vi "Write_Register.vi"(8 "error in (no error)":errorcluster, 9 "Value":u16, 10 "Address":u16 format="%x", 11 "Serial Config":T1={"Baud"=9600, "Flow Ctl"=0, "Parity"=0, "Address"=1, "VISA resource name"=""} {"Parity" items=["None", "Odd", "Even"]; "Flow Ctl" items=["None"]; "Baud" items=["4800"=4800, "9600"=9600, "19200"=19200, "38400"=38400]}) -> (0 "error out":errorcluster, 3 "Serial Config out":T1={"Baud"=9600, "Flow Ctl"=0, "Parity"=0, "Address"=0, "VISA resource name"=""} {"Parity" items=["None", "Odd", "Even"]; "Flow Ctl" items=["None"]; "Baud" items=["4800"=4800, "9600"=9600, "19200"=19200, "38400"=38400]})   [LabVIEW 2014, in "Omega CN9600 series.lvclass"]
uses:
  Omega CN9600 series.lvclass
  Serial_Config_Omega.ctl
  <vilib>/Utility/error.llb/Error Cluster From Error Code.vi
  <vilib>/ErrorRing/Error Ring.xnode
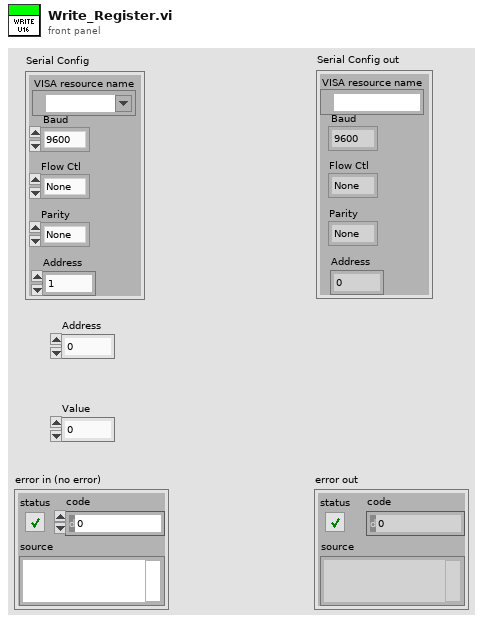
[diagram p1: front panel]
types:
  T1 = typedef "Omega CN9600 series.lvclass/Serial_Config_Omega.ctl" = cluster{"Baud":u32, "Flow Ctl":u16, "Parity":u16, "Address":u8, "VISA resource name":refnum<visa-resource-name>}
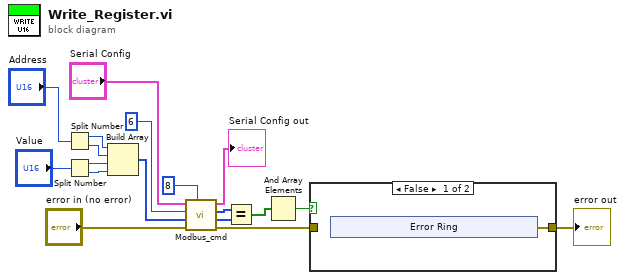
[diagram p0: block diagram]
diagram:
  n1 = Split Number(x="Address") -> (hi(x)=w12:u8, lo(x)=w11:u8)
  n2 = Split Number(x="Value") -> (hi(x)=w2:u8, lo(x)=w1:u8)
  n3 = Build Array(w12, w11, w2, w1) -> (w10:u8[])
  n4 = call "Modbus_cmd.vi"("Bytes to read"=u32 8, "error in (no error)"="error in (no error)", "Data"=w10, "Function"=u8 6, "Serial Config"="Serial Config") -> ("error out"=w4:errorcluster, "Cmd Sent"=w8:u8[], "Response"=w9:u8[], "Serial Config out"=→"Serial Config out":T1)  [unwired: 3 in]
  n5 = Equal?(x=w9, y=w8) -> (x = y?=w7:bool[])
  n6 = And Array Elements(Boolean array=w7) -> (logical AND=w6:bool)
  n7 = case shown="False" w6 {
    tunnel: [w19 w25] -> w5
    tunnel: w4 -> [_ w25]
    frame False {
      n8 = xnode "Error Ring"() -> ("error out"=w19:errorcluster)
    }
    frame True {
    }
  }
  "error out" <- w5
